vi "Update Current Execution Time.vi"(8 "error in (no error)":errorcluster, 10 "Current Execution Time (us)":u32, 11 "Execution Unit in":refnum<class "Execution Unit.lvclass">) -> (0 "error out":errorcluster, 3 "Execution Unit out":refnum<class "Execution Unit.lvclass">)   [LabVIEW 2020, in "Ballard MIL-STD-1553 Engine.lvlib" / "Interfaces.lvlib" / "Execution Unit.lvclass"]
uses:
  Execution Unit.lvclass
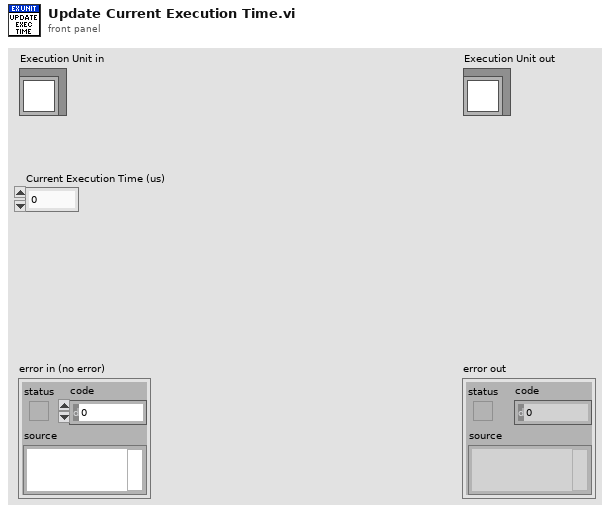
[diagram p1: front panel]
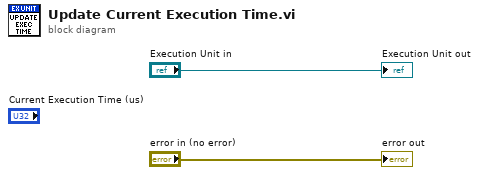
[diagram p0: block diagram]
diagram:
  "error out" <- "error in (no error)"
  "Execution Unit out" <- "Execution Unit in"
